vi "Main.vi"() -> ()   [LabVIEW 2015]
panel:
  in  "?":bool
  out "Numeric":u16
  in  "Select a Joystick":u16(ring) items=["Gamepad", "Extreme Joystick", "Other"]
  # "Please Mount Joystick Before Selecting"
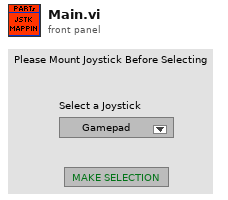
[diagram p1: front panel]
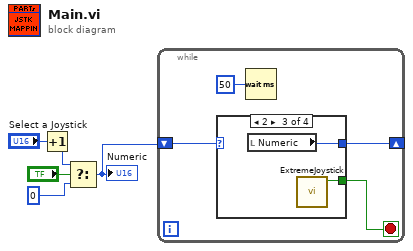
[diagram p0: block diagram]
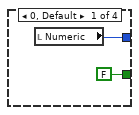
[diagram p2: hidden frame]
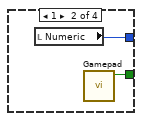
[diagram p3: hidden frame]
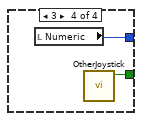
[diagram p4: hidden frame]
diagram:
  n1 = Increment(x="Select a Joystick") -> (x+1=w1:u16)
  n2 = Select(t=w1, s="?", f=u16 0) -> (s? t:f=w3:u16)
  "Numeric" <- w3
  n3 = while {
    shift-right: [w8] -> _
    shift-left: w3 -> [w9]
    stop <- w7 stop-if-true
    n4 = case shown="2" w9 {
      tunnel: [w11 w13 w15 w16] -> w8
      tunnel: [FALSE ("Stop") w12 w14 w17] -> w7
      frame 0, Default {
        n5 = local read "Numeric"() -> (w11:u16)
      }
      frame 1 {
        n6 = local read "Numeric"() -> (w13:u16)
        n7 = call "Gamepad.vi"() -> ("Stop"=w12:bool)  [unwired: 11 in]
      }
      frame 2 {
        n8 = local read "Numeric"() -> (w15:u16)
        n9 = call "ExtremeJoystick.vi"() -> ("Stop"=w14:bool)  [unwired: 11 in]
      }
      frame 3 {
        n10 = local read "Numeric"() -> (w16:u16)
        n11 = call "OtherJoystick.vi"() -> ("Stop"=w17:bool)  [unwired: 11 in]
      }
    }
    n12 = Wait (ms)(milliseconds to wait=u32 50) -> ()  [unwired: 1 out]
  }
